vi "combo analog digital io.vi"() -> ()   [LabVIEW 2018]
uses:
  <vilib>/DAQmx/read.llb/DAQmx Read (Analog 1D DBL NChan 1Samp).vi
  <vilib>/DAQmx/write.llb/DAQmx Write (Analog DBL 1Chan 1Samp).vi
  <vilib>/DAQmx/read.llb/DAQmx Read (Digital 1D Bool NChan 1Samp 1Line).vi
  <vilib>/DAQmx/write.llb/DAQmx Write (Digital 1D Bool NChan 1Samp 1Line).vi
  <vilib>/DAQmx/create/channels.llb/DAQmx Create Channel (DO-Digital Output).vi
  <vilib>/DAQmx/create/channels.llb/DAQmx Create Channel (DI-Digital Input).vi
  <vilib>/DAQmx/create/channels.llb/DAQmx Create Channel (AI-Voltage-Basic).vi
  <vilib>/DAQmx/create/channels.llb/DAQmx Create Channel (AO-Voltage-Basic).vi
  <vilib>/DAQmx/miscellaneous.llb/DAQmx Fill In Error Info.vi
  <vilib>/ptbypt/NI_PtbyPt.lvlib
panel:
  in  "Tab Control":enum32{"Operation", "Calibration", "Error"}(tab)
  out "Position":dbl format="%.4f"
  out "Load LBS":dbl
  out "Aux 3":dbl format="%.2f"
  out "Aux 2":dbl format="%.2f"
  out "Aux 1":dbl format="%.2f"
  out "C Amps":dbl format="%.2f"
  out "B Amps":dbl format="%.2f"
  out "A Amps":dbl format="%.2f"
  out "Tension":bool
  out "Compression":bool
  out "Load vs Postion":cluster{"mean":dbl, "mean":dbl}(graph)
  in  "stop":bool
  out "C Amps 2":dbl format="%.2f"
  out "B Amps 2":dbl format="%.2f"
  out "A Amps 2":dbl format="%.2f"
  in  "Phase C Bias":dbl
  in  "Phase C Scale":dbl=8.0 format="%#_13g"
  in  "Phase B Bias":dbl
  in  "Phase B Scale":dbl=8.0 format="%#_13g"
  in  "Phase A Bias":dbl
  in  "Phase A Scale":dbl=8.0 format="%#_13g"
  in  "Load Bias":dbl=-1.5
  in  "Load Scale":dbl=150.0 format="%#_13g"
  in  "Pos Bias":dbl=-0.005
  in  "Pos Scale":dbl=1.0 format="%#_13g"
  out "DAQ Output":dbl format="%.2f"
  out "Load Input":dbl format="%.2f"
  out "Air PSI":dbl format="%.2f"
  out "DC Amps":dbl format="%.2f"
  in  "Relay 4":bool
  in  "Relay 3":bool
  out "error out":errorcluster
  out "error out 3":errorcluster
  out "error out 4":errorcluster
  out "error out 5":errorcluster
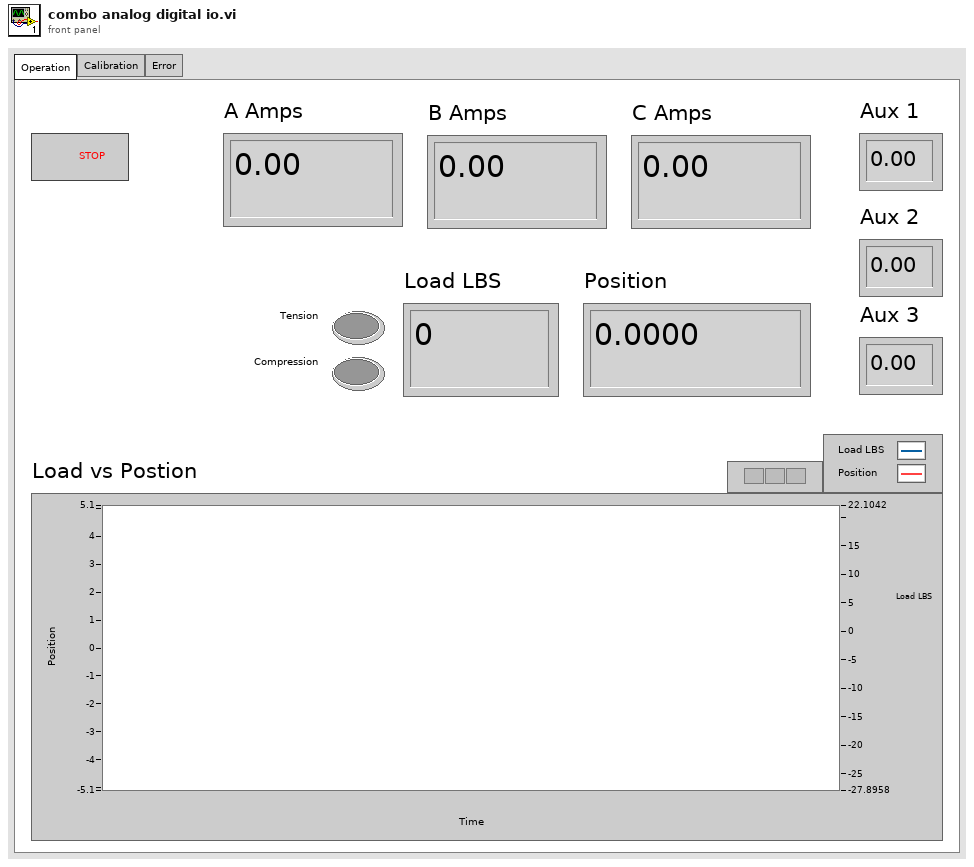
[diagram p1: front panel]
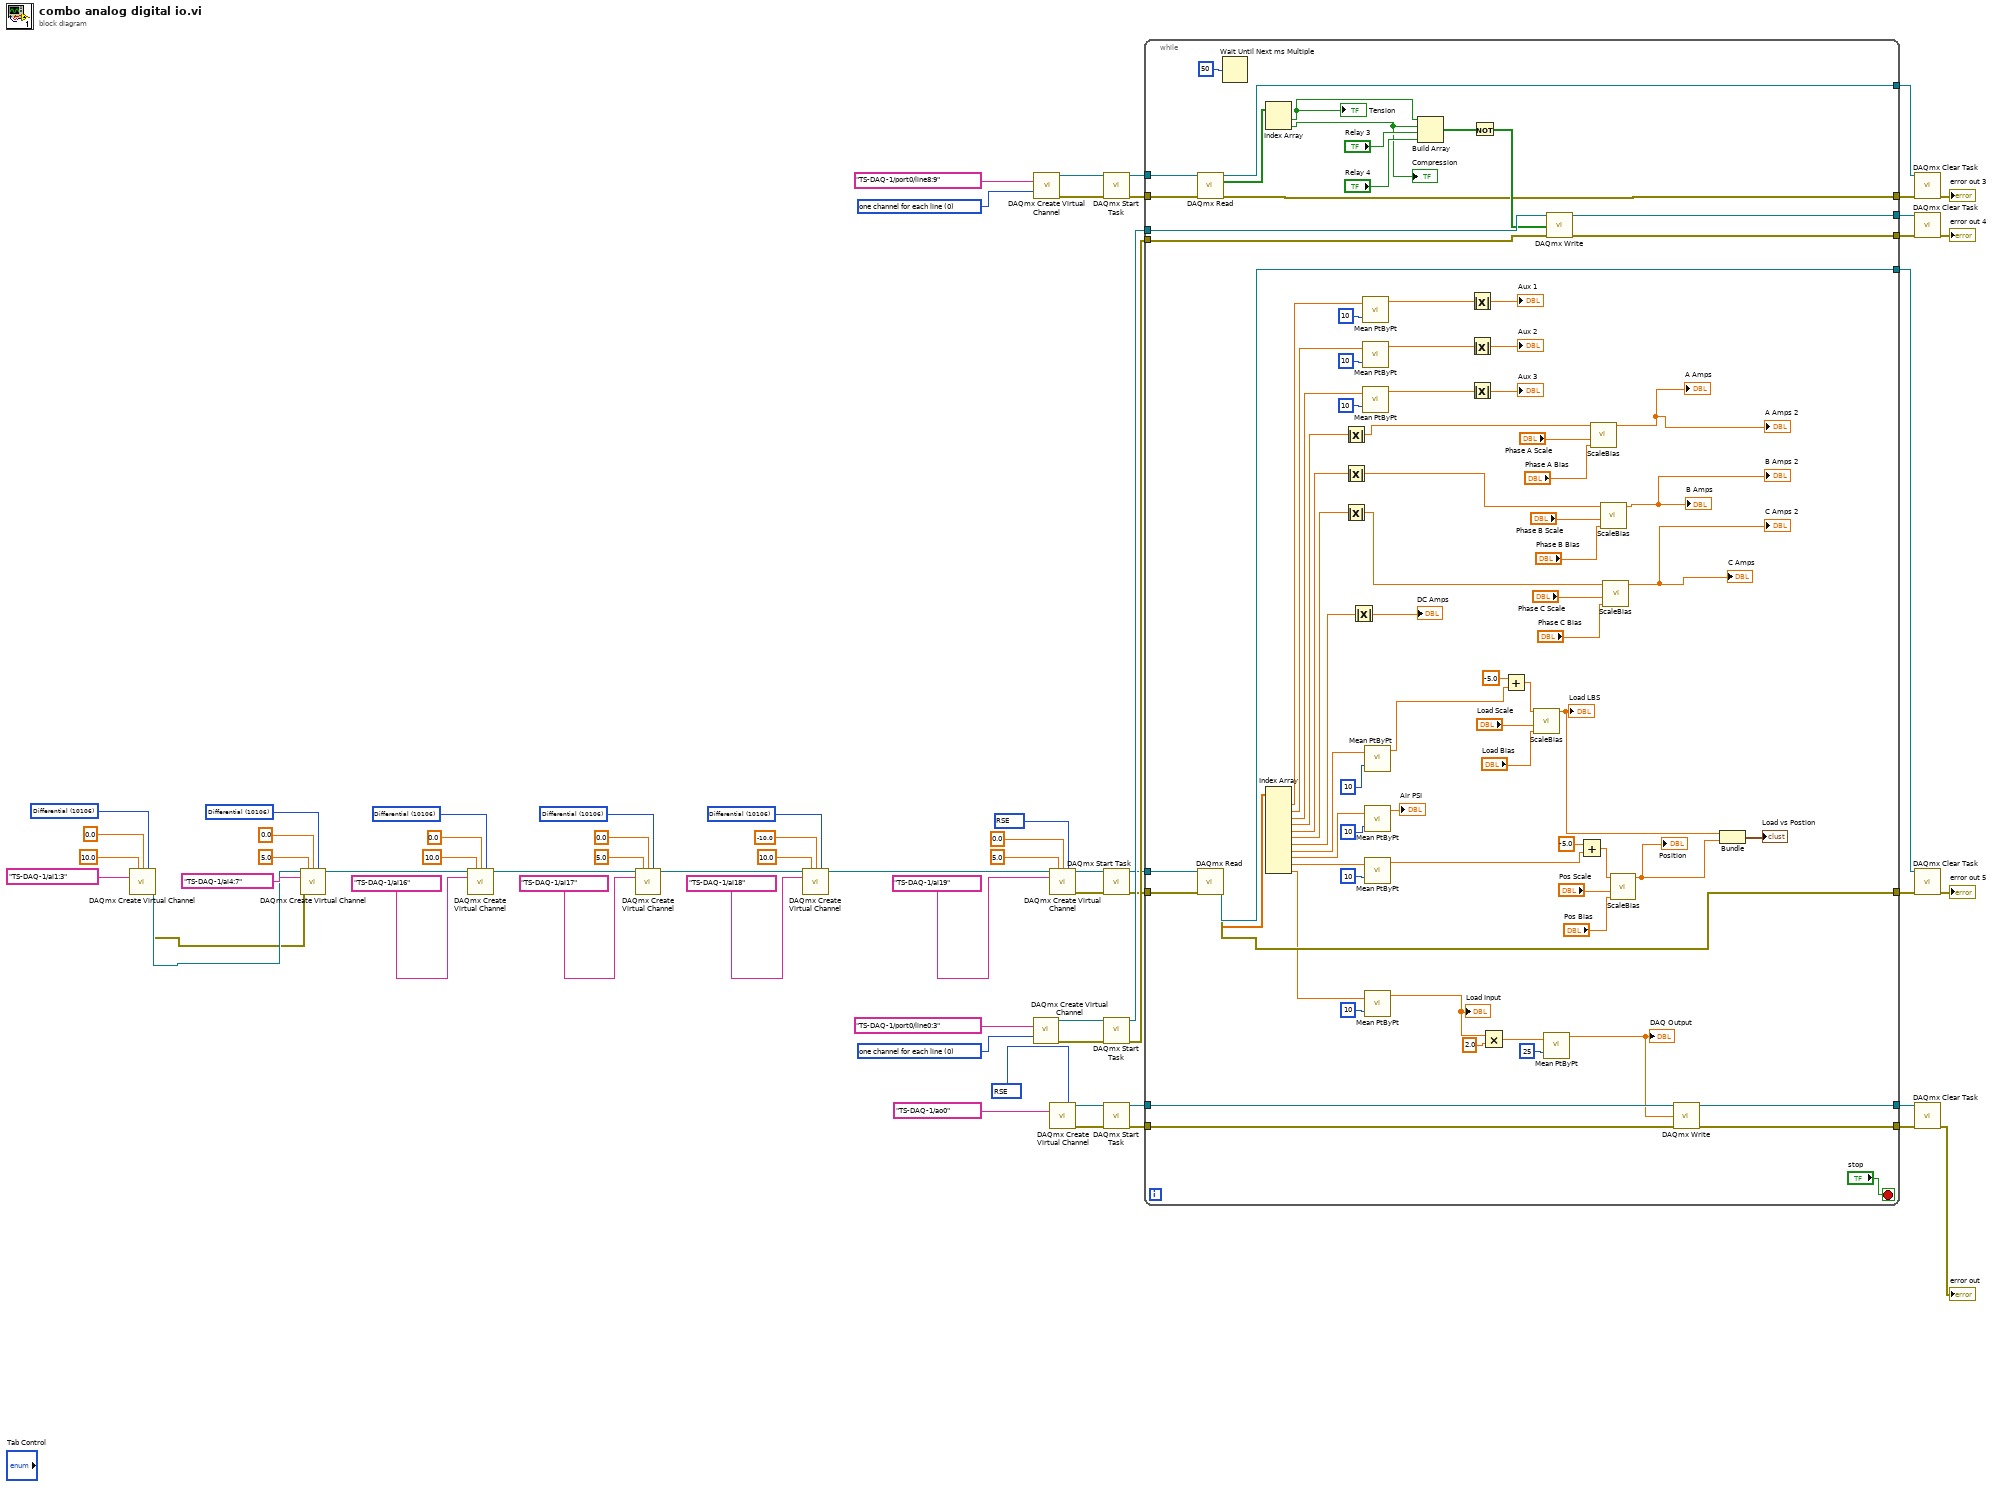
[diagram p0: block diagram]
diagram:
  w7 = 10106 items=["Default"=-1, "RSE"=10083, "NRSE"=10078, "Differential"=10106, "Pseudodifferential"=12529] ("input terminal configuration")
  w8 = 10106 items=["Default"=-1, "RSE"=10083, "NRSE"=10078, "Differential"=10106, "Pseudodifferential"=12529] ("input terminal configuration")
  w9 = 10106 items=["Default"=-1, "RSE"=10083, "NRSE"=10078, "Differential"=10106, "Pseudodifferential"=12529] ("input terminal configuration")
  w16 = 10083 items=["Default"=-1, "RSE"=10083, "Differential"=10106, "Pseudodifferential"=12529] ("output terminal configuration")
  w19 = 10083 items=["Default"=-1, "RSE"=10083, "NRSE"=10078, "Differential"=10106, "Pseudodifferential"=12529] ("input terminal configuration")
  w28 = 10106 items=["Default"=-1, "RSE"=10083, "NRSE"=10078, "Differential"=10106, "Pseudodifferential"=12529] ("input terminal configuration")
  w35 = 10106 items=["Default"=-1, "RSE"=10083, "NRSE"=10078, "Differential"=10106, "Pseudodifferential"=12529] ("input terminal configuration")
  w55 = 0 items=["one channel for each line", "one channel for all lines"] ("line grouping")
  w57 = 0 items=["one channel for each line", "one channel for all lines"] ("line grouping")
  n1 = call-poly <vilib>:"DAQmx Create Virtual Channel.vi"("maximum value"=10.0, "minimum value"=0.0, "input terminal configuration"=w28, "physical channels"=tag "TS-DAQ-1/ai1:3") -> ("task out"=w24:refnum<k21>, "error out"=w23:errorcluster)  [unwired: 10 in]
  n2 = call-poly <vilib>:"DAQmx Create Virtual Channel.vi"("task in"=w24, "maximum value"=5.0, "minimum value"=0.0, "input terminal configuration"=w35, "physical channels"=tag "TS-DAQ-1/ai4:7", "error in"=w23) -> ("task out"=w38:refnum<k21>)  [unwired: 8 in, 1 out]
  n3 = call-poly <vilib>:"DAQmx Create Virtual Channel.vi"("task in"=w38, "maximum value"=10.0, "minimum value"=0.0, "input terminal configuration"=w9, "physical channels"=tag "TS-DAQ-1/ai16") -> ("task out"=w15:refnum<k21>)  [unwired: 9 in, 1 out]
  n4 = call-poly <vilib>:"DAQmx Create Virtual Channel.vi"("task in"=w15, "maximum value"=5.0, "minimum value"=0.0, "input terminal configuration"=w8, "physical channels"=tag "TS-DAQ-1/ai17") -> ("task out"=w11:refnum<k21>)  [unwired: 9 in, 1 out]
  n5 = call-poly <vilib>:"DAQmx Create Virtual Channel.vi"("task in"=w11, "maximum value"=10.0, "minimum value"=-10.0, "input terminal configuration"=w7, "physical channels"=tag "TS-DAQ-1/ai18") -> ("task out"=w14:refnum<k21>)  [unwired: 9 in, 1 out]
  n6 = call-poly <vilib>:"DAQmx Create Virtual Channel.vi"("lines"=tag "TS-DAQ-1/port0/line0:3", "line grouping"=w57) -> ("task out"=w60:refnum<k21>, "error out"=w59:errorcluster)  [unwired: 12 in]
  n7 = call-poly <vilib>:"DAQmx Create Virtual Channel.vi"("lines"=tag "TS-DAQ-1/port0/line8:9", "line grouping"=w55) -> ("task out"=w54:refnum<k21>, "error out"=w51:errorcluster)  [unwired: 12 in]
  n8 = call-poly <vilib>:"DAQmx Create Virtual Channel.vi"("task in"=w14, "maximum value"=5.0, "minimum value"=0.0, "input terminal configuration"=w19, "physical channels"=tag "TS-DAQ-1/ai19") -> ("task out"=w22:refnum<k21>, "error out"=w21:errorcluster)  [unwired: 9 in]
  n9 = call-poly <vilib>:"DAQmx Create Virtual Channel.vi"("output terminal configuration"=w16, "physical channels"=tag "TS-DAQ-1/ao0") -> ("task out"=w46:refnum<k21>, "error out"=w45:errorcluster)  [unwired: 12 in]
  n10 = call <vilib>:"DAQmx Start Task.vi"("task/channels in"=w54, "error in"=w51) -> ("task out"=w53:refnum<k21>, "error out"=w50:errorcluster)  [unwired: 12 in]
  n11 = call <vilib>:"DAQmx Start Task.vi"("task/channels in"=w22, "error in"=w21) -> ("task out"=w37:refnum<k21>, "error out"=w36:errorcluster)  [unwired: 12 in]
  n12 = call <vilib>:"DAQmx Start Task.vi"("task/channels in"=w60, "error in"=w59) -> ("task out"=w64:refnum<k21>, "error out"=w63:errorcluster)  [unwired: 12 in]
  n13 = call <vilib>:"DAQmx Start Task.vi"("task/channels in"=w46, "error in"=w45) -> ("task out"=w44:refnum<k21>, "error out"=w43:errorcluster)  [unwired: 12 in]
  n14 = while {
    tunnel: w64 -> [w146]
    tunnel: [w145] -> w62
    tunnel: w63 -> [w143]
    tunnel: [w142] -> w61
    tunnel: w53 -> [w136]
    tunnel: [w135] -> w52
    tunnel: w50 -> [w134]
    tunnel: [w133] -> w49
    tunnel: [w131] -> w48
    tunnel: [w130] -> w47
    tunnel: w44 -> [w129]
    tunnel: w43 -> [w128]
    tunnel: w37 -> [w119]
    tunnel: w36 -> [w118]
    tunnel: [w117] -> w33
    tunnel: [w116] -> w32
    stop <- "stop" stop-if-true
    n15 = call-poly <vilib>:"DAQmx Read.vi"("task/channels in"=w136, "error in"=w134) -> ("task out"=w135:refnum<k21>, "data"=w132:bool[], "error out"=w133:errorcluster)  [unwired: 11 in]
    n16 = call-poly <vilib>:"DAQmx Read.vi"("task/channels in"=w119, "error in"=w118) -> ("task out"=w117:refnum<k21>, "data"=w115:dbl[], "error out"=w116:errorcluster)  [unwired: 11 in]
    n17 = Wait Until Next ms Multiple(millisecond multiple=u32 50) -> ()  [unwired: 1 out]
    n18 = Index Array(array=w132) -> (element #1=w122:bool, element #2=w123:bool)  [unwired: 2 in]
    "Compression" <- w123
    "Tension" <- w122
    n19 = Index Array(array=w115) -> (element #1=w104:dbl, element #2=w103:dbl, element #3=w102:dbl, element #4=w114:dbl, element #5=w113:dbl, element #6=w112:dbl, element #7=w111:dbl, element #8=w94:dbl, element #9=w96:dbl, element #10=w93:dbl, element #11=w97:dbl)  [unwired: 11 in]
    n20 = Absolute Value(x=w114) -> (abs(x)=w73:dbl)
    n21 = Absolute Value(x=w113) -> (abs(x)=w70:dbl)
    n22 = Absolute Value(x=w112) -> (abs(x)=w69:dbl)
    n23 = Absolute Value(x=w111) -> (abs(x)=→"DC Amps":dbl)
    n24 = call <vilib>:"Mean PtByPt.vi"("x"=w104, "sample length"=10) -> ("mean"=w105:dbl)  [unwired: 2 in, 1 out]
    n25 = call <vilib>:"Mean PtByPt.vi"("x"=w103, "sample length"=10) -> ("mean"=w106:dbl)  [unwired: 2 in, 1 out]
    n26 = call <vilib>:"Mean PtByPt.vi"("x"=w102, "sample length"=10) -> ("mean"=w107:dbl)  [unwired: 2 in, 1 out]
    n27 = call <vilib>:"Mean PtByPt.vi"("x"=w94, "sample length"=10) -> ("mean"=w87:dbl)  [unwired: 2 in, 1 out]
    n28 = call <vilib>:"Mean PtByPt.vi"("x"=w96, "sample length"=10) -> ("mean"=→"Air PSI":dbl)  [unwired: 2 in, 1 out]
    n29 = call <vilib>:"Mean PtByPt.vi"("x"=w93, "sample length"=10) -> ("mean"=w89:dbl)  [unwired: 2 in, 1 out]
    n30 = call <vilib>:"Mean PtByPt.vi"("x"=w97, "sample length"=10) -> ("mean"=w121:dbl)  [unwired: 2 in, 1 out]
    "Load Input" <- w121
    n31 = Build Array(w122, w123, "Relay 3", "Relay 4") -> (w138:bool[])
    n32 = Absolute Value(x=w105) -> (abs(x)=→"Aux 1":dbl)
    n33 = Absolute Value(x=w106) -> (abs(x)=→"Aux 2":dbl)
    n34 = Absolute Value(x=w107) -> (abs(x)=→"Aux 3":dbl)
    n35 = Not(x=w138) -> (.not. x?=w137:bool[])
    n36 = Multiply(x=w121, y=2.0) -> (x*y=w125:dbl)
    n37 = Add(x=-5.0 ("Load V Offset"), y=w87) -> (x+y=w77:dbl)
    n38 = call "ScaleBias.vi"("Input"=w77, "Scale"="Load Scale", "Bias"="Load Bias") -> ("Output"=w85:dbl)  [unwired: 6 in]
    "Load LBS" <- w85
    n39 = call <vilib>:"Mean PtByPt.vi"("x"=w125, "sample length"=25) -> ("mean"=w120:dbl)  [unwired: 2 in, 1 out]
    "DAQ Output" <- w120
    n40 = call-poly <vilib>:"DAQmx Write.vi"("task/channels in"=w146, "data"=w137, "error in"=w143) -> ("task out"=w145:refnum<k21>, "error out"=w142:errorcluster)  [unwired: 10 in, 1 out]
    n41 = Add(x=-5.0 ("Pos V Offset"), y=w89) -> (x+y=w74:dbl)
    n42 = call "ScaleBias.vi"("Input"=w73, "Scale"="Phase A Scale", "Bias"="Phase A Bias") -> ("Output"=→"A Amps" →"A Amps 2":dbl)  [unwired: 6 in]
    n43 = call "ScaleBias.vi"("Input"=w70, "Scale"="Phase B Scale", "Bias"="Phase B Bias") -> ("Output"=→"B Amps" →"B Amps 2":dbl)  [unwired: 6 in]
    n44 = call "ScaleBias.vi"("Input"=w69, "Scale"="Phase C Scale", "Bias"="Phase C Bias") -> ("Output"=→"C Amps" →"C Amps 2":dbl)  [unwired: 6 in]
    n45 = call "ScaleBias.vi"("Input"=w74, "Scale"="Pos Scale", "Bias"="Pos Bias") -> ("Output"=w78:dbl)  [unwired: 6 in]
    "Position" <- w78
    n46 = call-poly <vilib>:"DAQmx Write.vi"("task/channels in"=w129, "data"=w120, "error in"=w128) -> ("task out"=w131:refnum<k21>, "error out"=w130:errorcluster)  [unwired: 10 in, 1 out]
    n47 = Bundle("Output"=w85, "Output"=w78) -> (→"Load vs Postion":cluster{"Output":dbl, "Output":dbl})  [unwired: 1 in]
  }
  n48 = call <vilib>:"DAQmx Clear Task.vi"("task in"=w52, "error in"=w49) -> ("error out"=→"error out 3":errorcluster)  [unwired: 13 in]
  n49 = call <vilib>:"DAQmx Clear Task.vi"("task in"=w62, "error in"=w61) -> ("error out"=→"error out 4":errorcluster)  [unwired: 13 in]
  n50 = call <vilib>:"DAQmx Clear Task.vi"("task in"=w33, "error in"=w32) -> ("error out"=→"error out 5":errorcluster)  [unwired: 13 in]
  n51 = call <vilib>:"DAQmx Clear Task.vi"("task in"=w48, "error in"=w47) -> ("error out"=→"error out":errorcluster)  [unwired: 13 in]
